vi "DoorAccess - 複製.vi"() -> ()   [LabVIEW 2011]
uses:
  <vilib>/Platform/TimedLoop/XDataNode/timing_clust.ctl
  <vilib>/Platform/TimedLoop/XDataNode/nitl_modes.ctl
  <vilib>/Platform/TimedLoop/XDataNode/wakeup.ctl
  Variable/gSTOP.vi
  Routine/Queue/Alert.vi
  Routine/Queue/Card.vi
  Routine/DoorTread/Tread_03.vi
  Routine/DoorTread/Alerts.vi
  Routine/DoorTread/Tread_02.vi
  Routine/DoorTread/Tread_01.vi
  <vilib>/Platform/TimedLoop/XDataNode/XDataNode.xnode
  <vilib>/Platform/TimedLoop/XDataNode/XDNodeRunTimeDep.lvlib
panel:
  out "Warning":bool
  in  "En3":bool=TRUE
  in  "ID 3":u8=3
  in  "IP 3":string="192.168.1.128"
  in  "Port 3":u16=1621
  in  "Number 3":u8=3
  in  "stop":bool
  in  "ID 1":u8=1
  in  "IP 1":string="192.168.1.126"
  in  "Port 1":u16=1621
  in  "Number 1":u8=3
  in  "Number 2":u8=3
  in  "Port 2":u16=1621
  in  "IP 2":string="192.168.1.127"
  in  "ID 2":u8=2
  in  "En2":bool=TRUE
  out "Card Info":string="002001/22548:59693"
  out "Certificate":bool
  in  "En1":bool=TRUE
  in  "En0":bool
  in  "ID 0":u8
  in  "IP 0":string="localhost"
  in  "Port 0":u16=6341
  # "Door Access System v0.1\nDesigner : Ares.Chung"
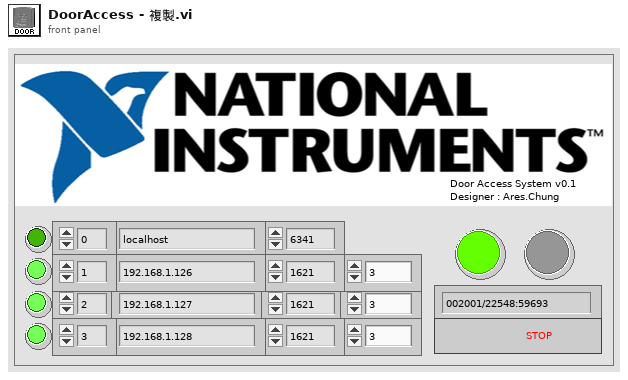
[diagram p1: front panel]
types:
  T1 = enum16{"Obtain", "Enqueue", "Dequeue", "Release"}
  T2 = typedef "XDNodeRunTimeDep.lvlib/timing_clust.ctl" = cluster{"Expected End [f-1]":u64, "Actual End [f-1]":u64, "Finished Late? [f-1]":bool, "Expected End [i-1]":u64, "Actual End [i-1]":u64, "Finished Late? [i-1]":bool, "Expected Start [i]":u64, "Actual Start [i]":u64, "Expected Start [f]":u64, "Actual Start [f]":u64, "Source Name":string, "Structure Name":string, "Period":i64, "Deadline":i64, "Offset":i64, "Start":i64, "Priority":i32, "Timeout":i32, "Mode":T3, "Wakeup Reason":T4, "Error":errorcluster, "Source Type":string, "Secondary Source Type":string, "Global End Time":u64, "Global Start Time":u64, "Frame Duration":u64, "Iteration Duration":u64, "Assigned CPU":i32, "I/O Scan Engine Mode":u32}
  T3 = typedef "XDNodeRunTimeDep.lvlib/nitl_modes.ctl" = enum32{"No Change", "Process missed periods, maintain original phase", "Discard missed periods, maintain original phase", "Process missed periods, ignore original phase", "Discard missed periods, ignore original phase"}
  T4 = typedef "XDNodeRunTimeDep.lvlib/wakeup.ctl" = enum32{"Normal", "Aborted", "Asynchronous wakeup", "Timing source error", "Timed loop error", "Timeout"}
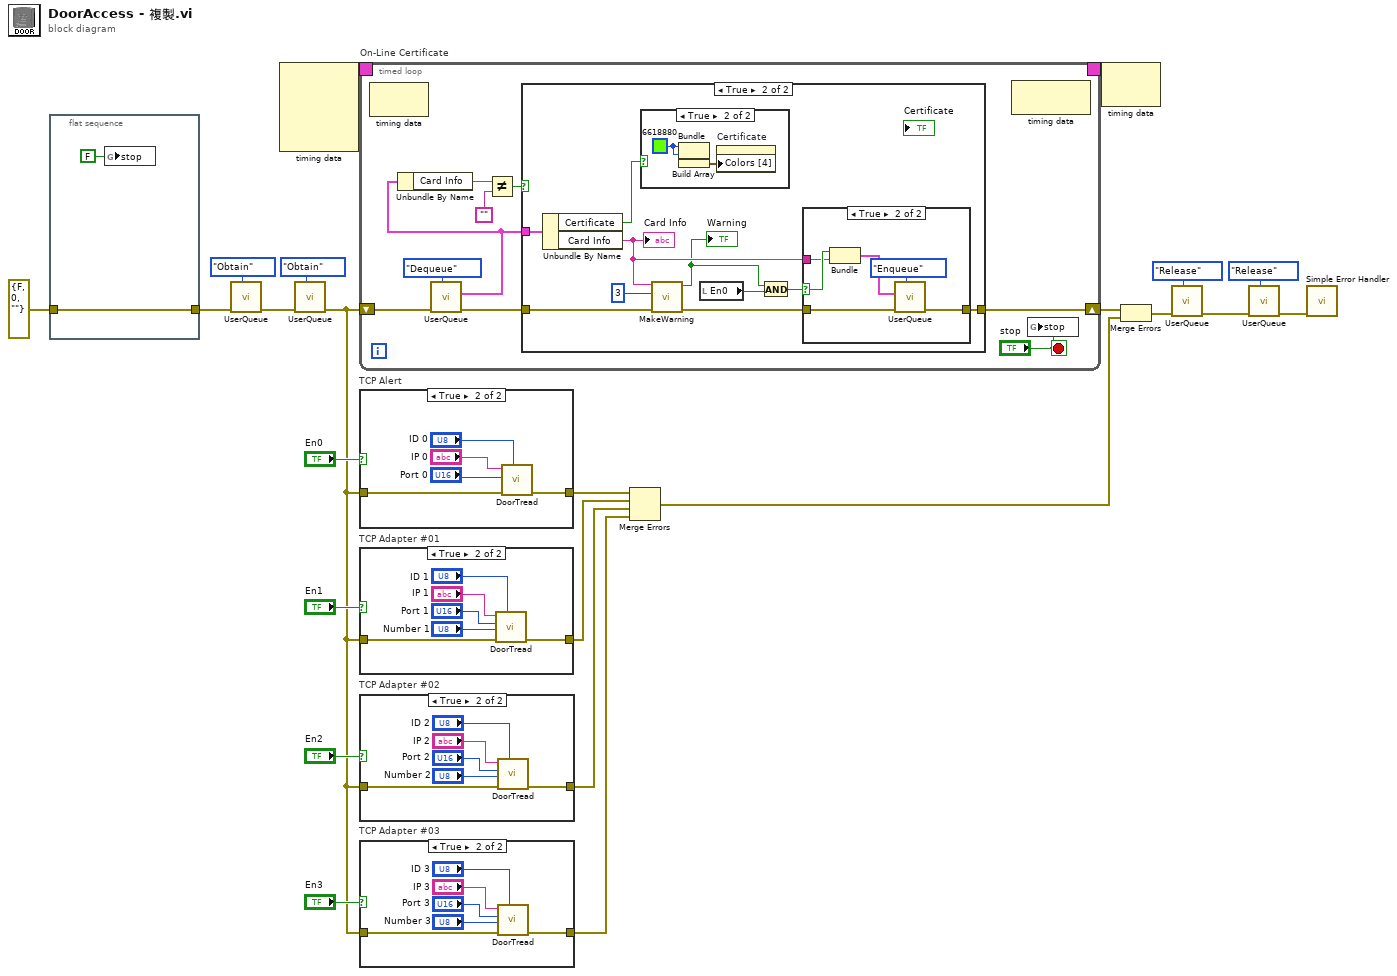
[diagram p0: block diagram]
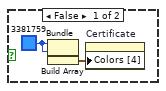
[diagram p5: hidden frame]
diagram:
  n1 = flat-sequence {
    tunnel: errorcluster {"status"=FALSE, "code"=0, "source"=""} ("error constant") -> [w24]
    tunnel: [w24] -> w5
    frame #0 {
      n2 = global write "gSTOP.vi" "stop"(FALSE ("stop")) -> ()
    }
  }
  n3 = call-poly "UserQueue.vi"("Mode"=T1."Obtain", "error in (no error)"=w5) -> ("error out"=w4:errorcluster)  [unwired: 8 in, 1 out]
  n4 = node-c288() -> (w13:T2)  [unwired: 4 in]
  n5 = call-poly "UserQueue.vi"("Mode"=T1."Obtain", "error in (no error)"=w4) -> ("error out"=w9:errorcluster)  [unwired: 8 in, 1 out]
  n6 = timed-loop "On-Line Certificate" {
    shift-right: [w29] -> w15
    shift-left: w9 -> [w33]
    timing: w13 -> [_]
    timing-out: [_] -> w12
    stop <- "stop" stop-if-true
    n7 = node-c288() -> ()  [unwired: 1 in, 1 out]
    n8 = call-poly "UserQueue.vi"("Mode"=T1."Dequeue", "error in (no error)"=w33) -> ("error out"=w30:errorcluster, "Queue Out"=w28:cluster{"Certificate":bool, "Card Info":string})  [unwired: 8 in]
    n9 = Unbundle By Name(w28) -> ("Card Info"=w32:string)
    n10 = Not Equal?(x=w32, y="") -> (x != y?=w31:bool)
    n11 = case shown="True" w31 {
      tunnel: w30 -> [w37 w45]
      tunnel: [w37 w43] -> w29
      tunnel: w28 -> [_ w47]
      frame False {
      }
      frame True {
        n12 = Unbundle By Name(w47) -> ("Certificate"=w46:bool, "Card Info"=w42:string)
        "Card Info" <- w42
        n13 = case shown="True" w46 {
          frame False {
            w57 = u32 3381759 ("Color Box")
            n14 = Bundle("Color Box"=w57, "Color Box"=w57) -> (w56:cluster{"Color Box":u32, "Color Box":u32})  [unwired: 1 in]
            n15 = Build Array(w56) -> (w55:cluster{"Color Box":u32, "Color Box":u32}[])
            n16 = property on="Certificate" class="Bool (strict)"("Colors [4]"=w55) -> ()  [unwired: 2 in, 2 out]
          }
          frame True {
            w60 = u32 6618880 ("Color Box")
            n17 = Bundle("Color Box"=w60, "Color Box"=w60) -> (w59:cluster{"Color Box":u32, "Color Box":u32})  [unwired: 1 in]
            n18 = Build Array(w59) -> (w58:cluster{"Color Box":u32, "Color Box":u32}[])
            n19 = property on="Certificate" class="Bool (strict)"("Colors [4]"=w58) -> ()  [unwired: 2 in, 2 out]
          }
        }
        n20 = call "MakeWarning.vi"("error in (no error)"=w45, "Setup"=u8 3, "String"=w42) -> ("error out"=w44:errorcluster, "Warning"=w39:bool)  [unwired: 7 in]
        "Warning" <- w39
        n21 = local read "En0"() -> (w40:bool)
        n22 = And(x=w39, y=w40) -> (x .and. y?=w38:bool)
        n23 = case shown="True" w38 {
          selector: w38 -> [_ w51]
          tunnel: w44 -> [w48 w53]
          tunnel: [w48 w52] -> w43
          tunnel: w42 -> [_ w50]
          frame False {
          }
          frame True {
            n24 = Bundle(w51, "Card Info"=w50) -> (w49:cluster{bool, "Card Info":string})  [unwired: 1 in]
            n25 = call-poly "UserQueue.vi"("Mode"=T1."Enqueue", "error in (no error)"=w53, "Queue In"=w49) -> ("error out"=w52:errorcluster)  [unwired: 7 in, 1 out]
          }
        }
      }
    }
    n26 = node-c288() -> ()  [unwired: 1 in, 1 out]
    n27 = global write "gSTOP.vi" "stop"("stop") -> ()
  }
  n28 = case "TCP Alert" shown="True" "En0" {
    tunnel: w9 -> [w61 w66]
    tunnel: [w61 w62] -> w11
    frame False {
    }
    frame True {
      n29 = call-poly "DoorTread.vi"("ID"="ID 0", "error in (no error)"=w66, "Port"="Port 0", "IP"="IP 0") -> ("error out"=w62:errorcluster)  [unwired: 7 in]
    }
  }
  n30 = case "TCP Adapter #01" shown="True" "En1" {
    tunnel: w9 -> [w67 w73]
    tunnel: [w67 w69] -> w17
    frame False {
    }
    frame True {
      n31 = call-poly "DoorTread.vi"("ID"="ID 1", "error in (no error)"=w73, "Number"="Number 1", "Port"="Port 1", "IP"="IP 1") -> ("error out"=w69:errorcluster)  [unwired: 6 in]
    }
  }
  n32 = case "TCP Adapter #02" shown="True" "En2" {
    tunnel: w9 -> [w74 w80]
    tunnel: [w74 w75] -> w16
    frame False {
    }
    frame True {
      n33 = call-poly "DoorTread.vi"("ID"="ID 2", "error in (no error)"=w80, "Number"="Number 2", "Port"="Port 2", "IP"="IP 2") -> ("error out"=w75:errorcluster)  [unwired: 6 in]
    }
  }
  n34 = case "TCP Adapter #03" shown="True" "En3" {
    tunnel: w9 -> [w81 w87]
    tunnel: [w81 w82] -> w8
    frame False {
    }
    frame True {
      n35 = call-poly "DoorTread.vi"("ID"="ID 3", "error in (no error)"=w87, "Number"="Number 3", "Port"="Port 3", "IP"="IP 3") -> ("error out"=w82:errorcluster)  [unwired: 6 in]
    }
  }
  n36 = Merge Errors(w11, w17, w16, w8) -> (w14:errorcluster)
  n37 = node-c288(w12) -> ()  [unwired: 1 out]
  n38 = Merge Errors(w15, w14) -> (w18:errorcluster)
  n39 = call-poly "UserQueue.vi"("Mode"=T1."Release", "error in (no error)"=w18) -> ("error out"=w2:errorcluster)  [unwired: 8 in, 1 out]
  n40 = call-poly "UserQueue.vi"("Mode"=T1."Release", "error in (no error)"=w2) -> ("error out"=w1:errorcluster)  [unwired: 8 in, 1 out]
  n41 = call <vilib>:"Simple Error Handler.vi"("error in (no error)"=w1) -> ()  [unwired: 4 in, 5 out]
